vi "calculator.vi"() -> ()   [LabVIEW 2019]
panel:
  in  "Tab Control":enum32{"Calculator"}(tab)
  out "If Y is Divided by 0":bool
  in  "?":bool
  out "Result":dbl
  in  "X":dbl
  in  "Y":dbl
  in  "Toggle":bool
  # "No Light:\nDivision"
  # "Green Light: \nSubtraction"
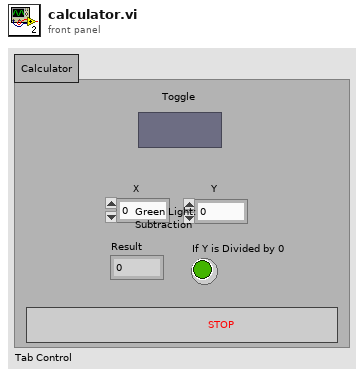
[diagram p1: front panel]
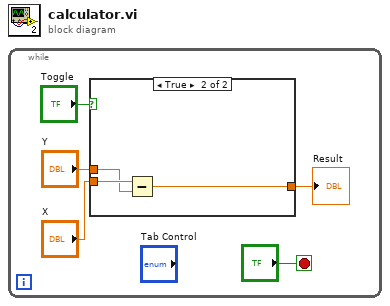
[diagram p0: block diagram]
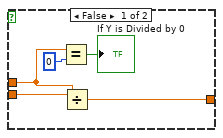
[diagram p2: hidden frame]
diagram:
  n1 = while {
    stop <- "?" stop-if-true
    n2 = case shown="True" "Toggle" {
      tunnel: "X" -> [w10 w13]
      tunnel: "Y" -> [w8 w12]
      tunnel: [w9 w11] -> w2
      frame False {
        n3 = Equal?(x=w8, y=0) -> (x = y?=→"If Y is Divided by 0":bool)
        n4 = Divide(x=w10, y=w8) -> (x/y=w9:dbl)
      }
      frame True {
        n5 = Subtract(x=w13, y=w12) -> (x-y=w11:dbl)
      }
    }
    "Result" <- w2
  }
